vi "Startup.vi"() -> ()   [LabVIEW 2011]
uses:
  Lib/JLinkARM.lvlib
panel:
  out "not successful":bool
  out "Connect successful":bool
  out "Output":string
  out "String":string
  in  "IP":bool
  in  "IP:":string
  in  "CLOSE":bool
  in  "Serial Number:":dbl
  in  "Interface:":i32(listbox)
  in  "Speed [kHz]:":dbl
  in  "Device:":string
  in  "stop":bool
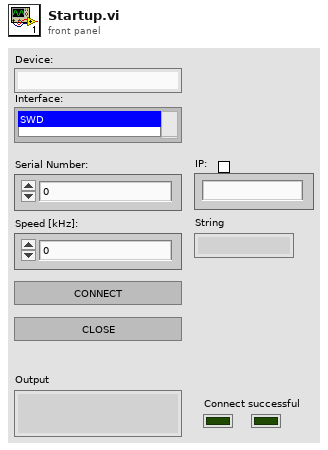
[diagram p1: front panel]
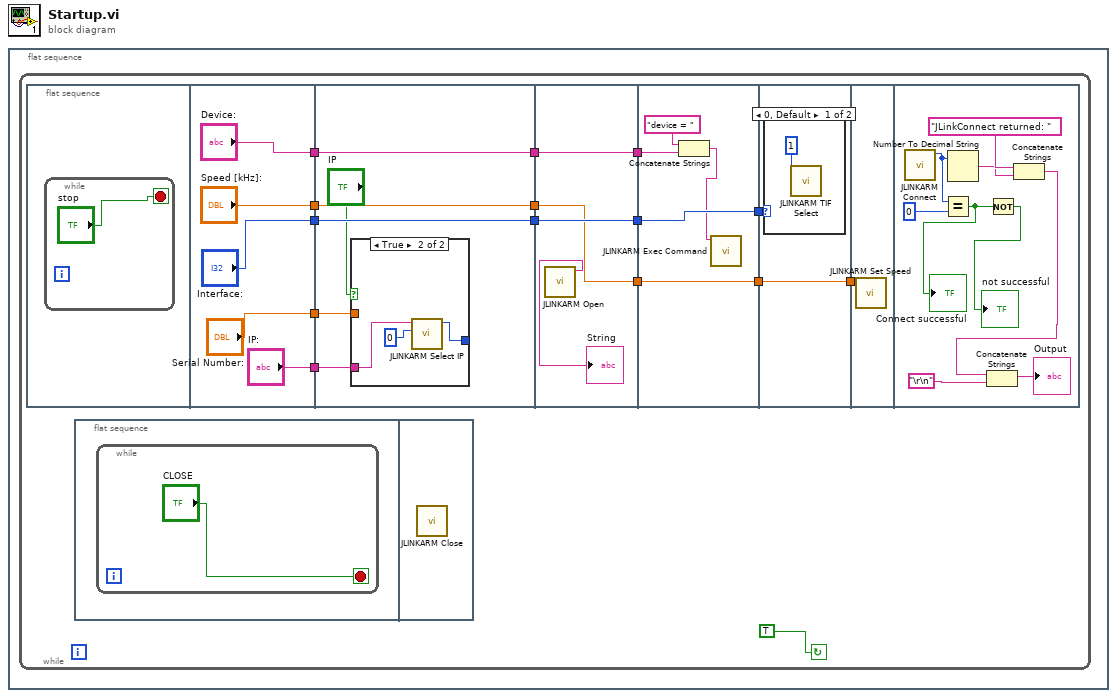
[diagram p0: block diagram]
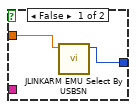
[diagram p2: hidden frame]
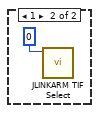
[diagram p3: hidden frame]
diagram:
  n1 = flat-sequence {
    frame #0 {
      n2 = while {
        stop <- TRUE continue-if-true
        n3 = flat-sequence {
          tunnel: ["Serial Number:"] -> w14
          tunnel: ["Interface:"] -> w10
          tunnel: ["Speed [kHz]:"] -> w9
          tunnel: ["Device:"] -> w2
          tunnel: ["IP:"] -> w1
          tunnel: w14 -> [w23]
          tunnel: [w28] -> w11
          tunnel: w10 -> [w28]
          tunnel: w9 -> [w27]
          tunnel: [w27] -> w8
          tunnel: [w26] -> w3
          tunnel: w2 -> [w26]
          tunnel: w1 -> [w24]
          tunnel: [w37] -> w12
          tunnel: w11 -> [w37]
          tunnel: w8 -> [w36]
          tunnel: [w36] -> w7
          tunnel: [w35] -> w4
          tunnel: w3 -> [w35]
          tunnel: [w42] -> w13
          tunnel: w12 -> [w42]
          tunnel: w7 -> [w41]
          tunnel: [w41] -> w6
          tunnel: w4 -> [w39]
          tunnel: w13 -> [w44]
          tunnel: w6 -> [w43]
          tunnel: [w43] -> w5
          tunnel: w5 -> [w47]
          frame #0 {
            n4 = while {
              stop <- "stop" stop-if-true
            }
          }
          frame #1 {
          }
          frame #2 {
            n5 = case shown="True" "IP" {
              tunnel: w24 -> [_ w33]
              tunnel: w23 -> [w30 _]
              tunnel: [w29 w31] -> _
              frame False {
                n6 = call "JLINKARM EMU Select By USBSN.vi"("SerialNo"=w30) -> ("function return"=w29:i32)  [unwired: 10 in]
              }
              frame True {
                n7 = call "JLINKARM Select IP.vi"("Port"=0, "sHost"=w33) -> ("function return"=w31:i8)  [unwired: 9 in]
              }
            }
          }
          frame #3 {
            n8 = call "JLINKARM Open.vi"() -> ("function return"=→"String":string)  [unwired: 11 in]
          }
          frame #4 {
            n9 = Concatenate Strings("device = ", w39) -> (w38:string)
            n10 = call "JLINKARM Exec Command.vi"("pIn"=w38) -> ()  [unwired: 9 in, 2 out]
          }
          frame #5 {
            n11 = case shown="0, Default" w44 {
              frame 0, Default {
                n12 = call "JLINKARM TIF Select.vi"("Interface"=1) -> ()  [unwired: 10 in, 1 out]
              }
              frame 1 {
                n13 = call "JLINKARM TIF Select.vi"("Interface"=0) -> ()  [unwired: 10 in, 1 out]
              }
            }
          }
          frame #6 {
            n14 = call "JLINKARM Set Speed.vi"("Speed"=w47) -> ()  [unwired: 11 in]
          }
          frame #7 {
            n15 = call "JLINKARM Connect.vi"() -> ("function return"=w51:i32)  [unwired: 11 in]
            n16 = Equal?(x=w51, y=0) -> (x = y?=w50:bool)
            "Connect successful" <- w50
            n17 = Number To Decimal String(number=w51) -> (decimal integer string=w53:string)  [unwired: 1 in]
            n18 = Not(x=w50) -> (.not. x?=→"not successful":bool)
            n19 = Concatenate Strings("JLinkConnect returned: ", w53) -> (w48:string)
            n20 = Concatenate Strings(w48, "\r\n") -> (→"Output":string)
          }
        }
        n21 = flat-sequence {
          frame #0 {
            n22 = while {
              stop <- "CLOSE" stop-if-true
            }
          }
          frame #1 {
            n23 = call "JLINKARM Close.vi"() -> ()  [unwired: 12 in]
          }
        }
      }
    }
  }
